vi "get all sub folders list which has files.vi"(11 "Folder Path":path=path "D:/Library/Mobile Repository/Sam Mobile") -> (3 "All Folders":path[](array[path]))   [LabVIEW 2023]
panel:
  out "no of folders with valid files":i32
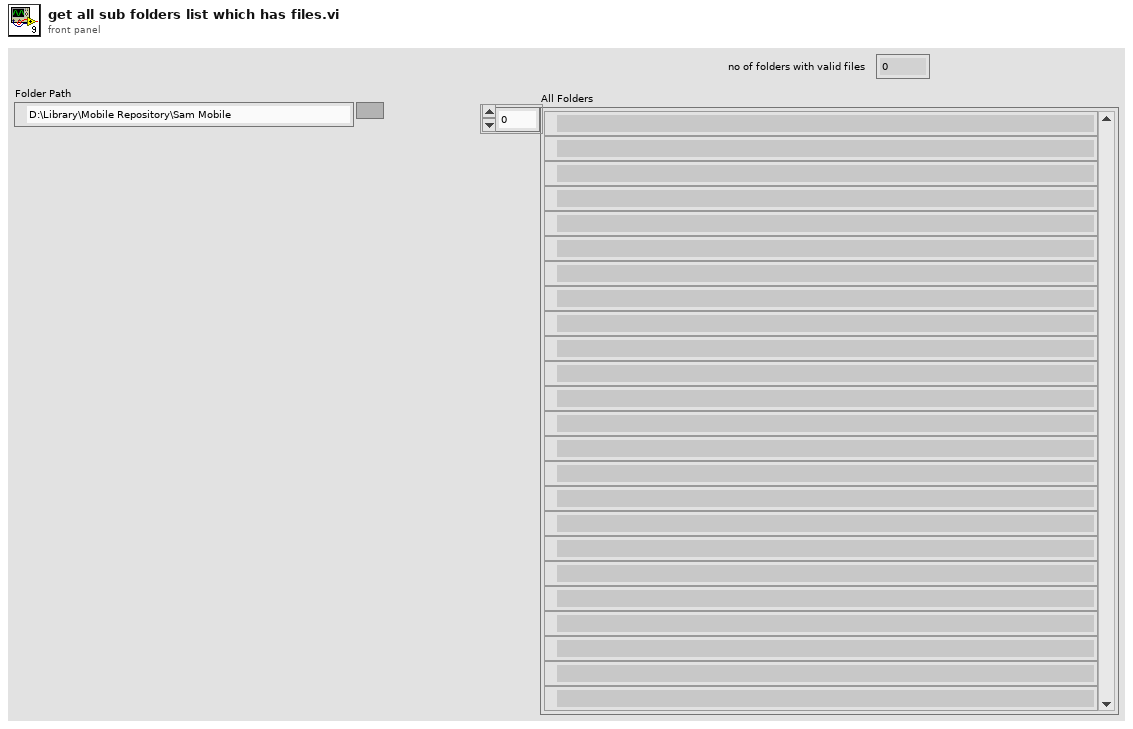
[diagram p1: front panel]
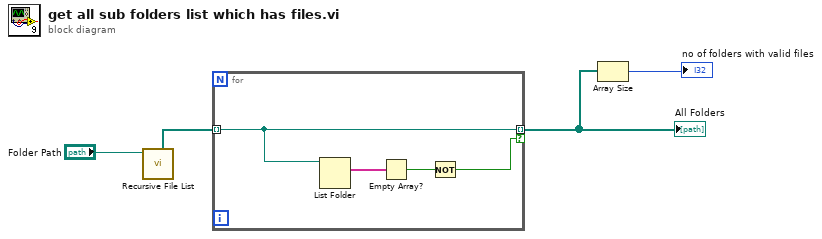
[diagram p0: block diagram]
diagram:
  n1 = call <vilib>:"Recursive File List.vi"("Folder Path"="Folder Path") -> ("All Folders"=w3:path[])  [unwired: 6 in, 4 out]
  n2 = for {
    tunnel: w3 -> [w8] mode=indexing
    tunnel: [w8] -> w2 mode=indexing if=w5
    n3 = List Folder(path=w8) -> (filenames=w7:string[])  [unwired: 3 in, 3 out]
    n4 = Empty Array?(array=w7) -> (empty?=w6:bool)
    n5 = Not(x=w6) -> (.not. x?=w5:bool)
  }
  "All Folders" <- w2
  n6 = Array Size(array=w2) -> (size(s)=→"no of folders with valid files":i32)
